vi "Send File.vi"(0 "TargetItem":refnum<vi>, 1 "Host Base Path":path, 2 "Filename":string, 3 "Error In":errorcluster) -> (8 "Target File":path, 10 "Error Out":errorcluster)   [LabVIEW 2023]
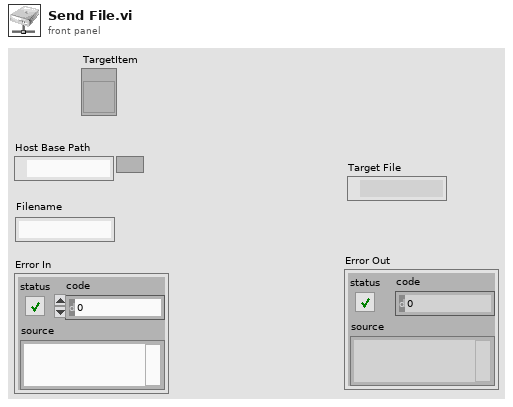
[diagram p1: front panel]
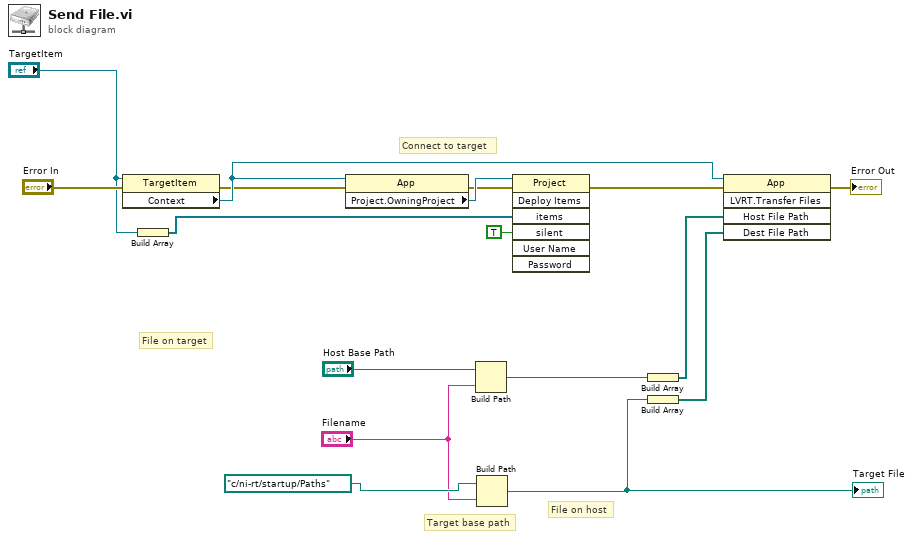
[diagram p0: block diagram]
diagram:
  # "Target base path"
  # "File on host"
  # "Connect to target"
  # "File on target"
  n1 = property class="TargetItem"(reference="TargetItem", error in="Error In") -> (error out=w7:errorcluster, "Context"=w10:refnum<vi>)  [unwired: 1 out]
  n2 = Build Array("TargetItem") -> (w4:refnum<vi>[])
  n3 = property class="App"(reference=w10, error in=w7) -> (error out=w6:errorcluster, "Project.OwningProject"=w9:refnum<vi>)  [unwired: 1 out]
  n4 = Build Path(base path="Host Base Path", name or relative path="Filename") -> (appended path=w2:path)
  n5 = Build Path(base path=path "c:/ni-rt/startup/Paths" ("Target Base Path"), name or relative path="Filename") -> (appended path=w15:path)
  "Target File" <- w15
  n6 = invoke class="Project" method="Deploy Items"(reference=w9, error in=w6, "items"=w4, "silent"=TRUE ("Silent")) -> (error out=w8:errorcluster)  [unwired: 3 in, 6 out]
  n7 = Build Array(w2) -> (w17:path[])
  n8 = Build Array(w15) -> (w16:path[])
  n9 = invoke class="App" method="LVRT.Transfer Files"(reference=w10, error in=w8, "Host File Path"=w17, "Dest File Path"=w16) -> (error out=→"Error Out":errorcluster)  [unwired: 1 in, 4 out]
